vi "Sample_Scan_Pause_Exe.vi"(5 "waiting time (ms)":u32, 6 "Spacing (t) / Long Side (f)":bool, 7 "Scan Mode":T2 caption="Scan Settings" items=["Mode 1", "Mode 2", "Reversed 1", "Reversed 2"], 8 "error in":errorcluster, 9 "velocity cluster":T1, 10 "Position Array":i32[](array[numeric]), 11 "VISA resource name":refnum<visa-resource-name>) -> (0 "error out":errorcluster={"status"=FALSE, "code"=1073676294, "source"="VISA Read in write_read.vi"}, 1 "velocity cluster out":T1, 2 "Position Array out":i32[](array[numeric]), 3 "VISA ressource out":refnum<visa-resource-name>, 4 "Move Motor":u16)   [LabVIEW 2018]
uses:
  Scan Mode.ctl
  MCode_LV_86/Set Parameter.ctl
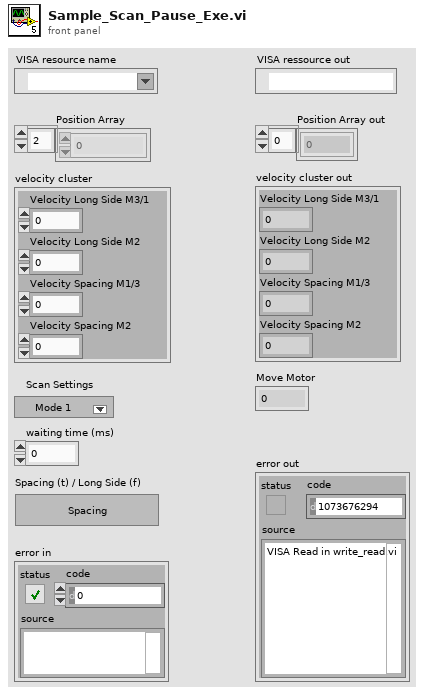
[diagram p1: front panel]
types:
  T1 = cluster{"Velocity Long Side M3/1":dbl, "Velocity Long Side M2":dbl, "Velocity Spacing M1/3":dbl, "Velocity Spacing M2":dbl}
  T2 = typedef "Scan Mode.ctl" = u16
  T3 = typedef "Set Parameter.ctl" = enum16{"Acceleration (A)", "Baud Rate (BD)", "Counter 1 (C1)", "Counter 2 (C2)", "Control C Software Reset (CE)", "Check Sum Enable (CK)", "Clock Mode (CM)", "Clock Mode Ratio (CR)", "Clock Mode Out Step Width (CW)", "Deceleration (D)", "Digital Filtering, Input 1 (D1)", "Digital Filtering, Input 2 (D2)", "Digital Filtering, Input 3 (D3)", "Digital Filtering, Input 4 (D4)", "Digital Filtering, Input 5 (D5)", "Digital Filtering, Input 9 (D9)", "Digital Filtering, Input 10 (D10)", "Digital Filtering, Input 11 (D11)", "Digital Filtering, Input 12 (D12)", "Deadband (DB)", "Decrement Variable (DC)", "Enable/Disable Drive (DE)", "Device Name (DN)", "End Program Execution (E)", "Encoder Function Enable (EE)", "Error Flag (EF)", "Encoder Lines (EL)", "Echo Mode (EM)", "Error Value (ER)", "Escape (ES)", "Execute Program at Address (EX)", "Firmware Version (VR)", "Hold (H)", "Hold Current (HC)", "Hold Current Delay Time (HI)", "Home to Encoder Index (HM)", "Home to Home Switch (HT)", "Increment Variable (IC)", "Initialize Parameters to NVM (IP)", "Input into Variable (IV)", "Jog Enable (JE)", "Limit Stop Mode (LM)", "Move Absolute (MA)", "Move Relative (MR)", "MicroStepping Select (MS)", "Motor Settling Delay Time (MT)", "Moving [Flag] (MV)", "Output 1 (O1)", "Output 2 (O2)", "Output 3 (O3)", "Output 4 (O4)", "Output 9 (O9)", "Output 10 (O10)", "Output 11 (O11)", "Output 12 (O12)", "Output High Byte (9-12) (OH)", "Output Low Byte (1-4) (OL)", "Output Total (1-4 and 9-12) (OT)", "Position (P)", "Position Maintenance (PM)", "Party Mode (PY)", "Register 1 (R1)", "Register 2 (R2)", "Register 3 (R3)", "Register 4 (R4)", "Reset Error(\\03)", "Run Current (RC)", "Stall Factor (SF)", "Slew (SL)", "Stall Mode Set (SM)", "Upgrade Firmware (UG)", "Velocity Initial (VI)", "Velocity Maximum (VM)", "Current1 (I1)", "Current2 (I2)", "Current3 (I3)", "Current4 (I4)", "Current5 (I5)", "Current6 (I6)", "Save (S)"}
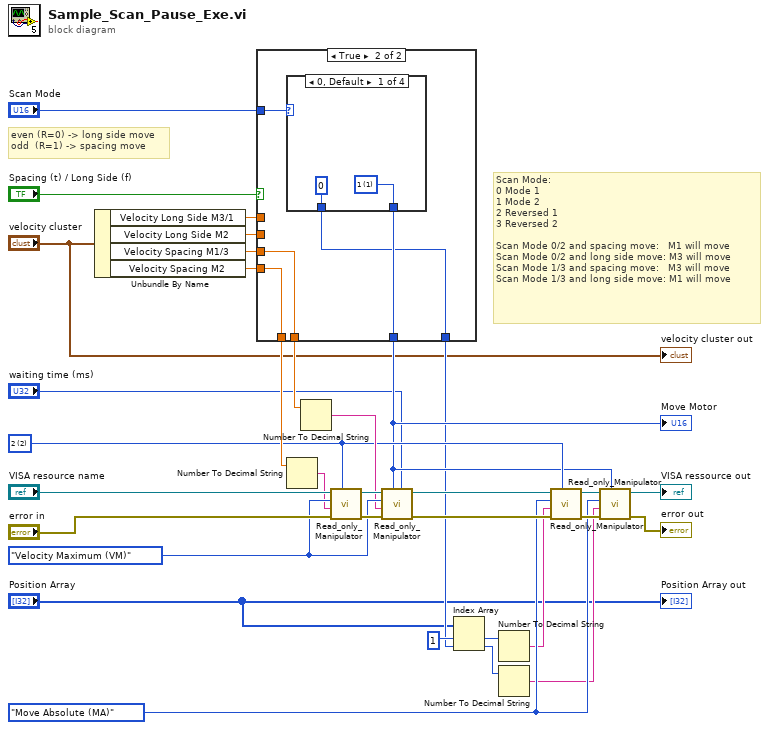
[diagram p0: block diagram]
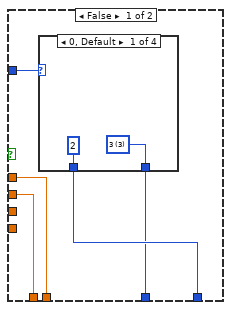
[diagram p2: hidden frame]
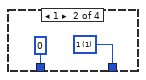
[diagram p3: hidden frame]
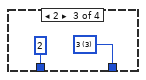
[diagram p4: hidden frame]
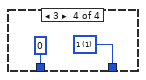
[diagram p5: hidden frame]
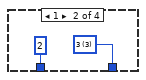
[diagram p6: hidden frame]
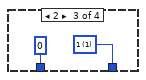
[diagram p7: hidden frame]
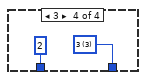
[diagram p8: hidden frame]
diagram:
  w10 = u16 2 items=["none", "1", "2", "3", "4", "all"] ("Motor")
  w21 = Set_Parameter."Move Absolute (MA)" ("Command")
  w22 = Set_Parameter."Velocity Maximum (VM)" ("Command")
  # "Scan Mode:\n0 Mode 1\n1 Mode 2\n2 Reversed 1\n3 Reversed 2\n\nScan Mode 0/2 and spacing move:   M1 will move\nScan Mode 0/2 and long side move: M3 will move\nScan Mode 1/3 and spacing move:   M3 will move\nScan Mode 1/3 and long side move: M1 will move"
  # "even (R=0) -> long side move\nodd  (R=1) -> spacing move"
  n1 = Unbundle By Name("velocity cluster") -> ("Velocity Long Side M3/1"=w19:dbl, "Velocity Long Side M2"=w18:dbl, "Velocity Spacing M1/3"=w17:dbl, "Velocity Spacing M2"=w16:dbl)
  n2 = case shown="True" "Spacing (t) / Long Side (f)" {
    tunnel: w19 -> [w37 _]
    tunnel: w18 -> [w38 _]
    tunnel: w17 -> [_ w50]
    tunnel: w16 -> [_ w49]
    tunnel: "Scan Mode" -> [w36 w51]
    tunnel: [w37 w50] -> w12
    tunnel: [w38 w49] -> w14
    tunnel: [w34 w48] -> w9
    tunnel: [w35 w47] -> w6
    frame False {
      n3 = case shown="0, Default" w36 {
        tunnel: [w40 w41 w44 w45] -> w34
        tunnel: [2 ("index") 0 ("index") 2 ("index") 0 ("index")] -> w35
        frame 0, Default {
          w40 = u16 3 items=["none", "1", "2", "3", "4", "all"] ("Motor")
        }
        frame 1 {
          w41 = u16 1 items=["none", "1", "2", "3", "4", "all"] ("Motor")
        }
        frame 2 {
          w44 = u16 3 items=["none", "1", "2", "3", "4", "all"] ("Motor")
        }
        frame 3 {
          w45 = u16 1 items=["none", "1", "2", "3", "4", "all"] ("Motor")
        }
      }
    }
    frame True {
      n4 = case shown="0, Default" w51 {
        tunnel: [w53 w54 w57 w58] -> w48
        tunnel: [0 ("index") 2 ("index") 0 ("index") 2 ("index")] -> w47
        frame 0, Default {
          w53 = u16 1 items=["none", "1", "2", "3", "4", "all"] ("Motor")
        }
        frame 1 {
          w54 = u16 3 items=["none", "1", "2", "3", "4", "all"] ("Motor")
        }
        frame 2 {
          w57 = u16 1 items=["none", "1", "2", "3", "4", "all"] ("Motor")
        }
        frame 3 {
          w58 = u16 3 items=["none", "1", "2", "3", "4", "all"] ("Motor")
        }
      }
    }
  }
  "Move Motor" <- w9
  n5 = Number To Decimal String(number=w14) -> (decimal integer string=w13:string)  [unwired: 1 in]
  n6 = Number To Decimal String(number=w12) -> (decimal integer string=w11:string)  [unwired: 1 in]
  n7 = call "Read_only_Manipulator.vi"("Motor"=w10, "error in (no error)"="error in", "Value"=w13, "Command"=w22, "VISA resource name"="VISA resource name") -> ("error out"=w29:errorcluster, "VISA ressource out"=w32:refnum<visa-resource-name>)  [unwired: 3 in, 2 out]
  n8 = call "Read_only_Manipulator.vi"("waiting time (ms)"="waiting time (ms)", "Motor"=w9, "error in (no error)"=w29, "Value"=w11, "Command"=w22, "VISA resource name"=w32) -> ("error out"=w28:errorcluster, "VISA ressource out"=w31:refnum<visa-resource-name>)  [unwired: 2 in, 2 out]
  n9 = Index Array(array="Position Array", index #1=1 ("index"), index #2=w6) -> (element #1=w8:i32, element #2=w5:i32)
  n10 = Number To Decimal String(number=w8) -> (decimal integer string=w7:string)  [unwired: 1 in]
  n11 = Number To Decimal String(number=w5) -> (decimal integer string=w4:string)  [unwired: 1 in]
  n12 = call "Read_only_Manipulator.vi"("Motor"=w10, "error in (no error)"=w28, "Value"=w7, "Command"=w21, "VISA resource name"=w31) -> ("error out"=w27:errorcluster, "VISA ressource out"=w30:refnum<visa-resource-name>)  [unwired: 3 in, 2 out]
  n13 = call "Read_only_Manipulator.vi"("Motor"=w9, "error in (no error)"=w27, "Value"=w4, "Command"=w21, "VISA resource name"=w30) -> ("error out"=→"error out":errorcluster, "VISA ressource out"=→"VISA ressource out":refnum<visa-resource-name>)  [unwired: 3 in, 2 out]
  "Position Array out" <- "Position Array"
  "velocity cluster out" <- "velocity cluster"
